vi "simulation.vi"() -> ()   [LabVIEW 2020]
uses:
  <vilib>/DAQmx/write.llb/DAQmx Write (Digital Bool 1Line 1Point).vi
  <vilib>/DAQmx/create/channels.llb/DAQmx Create Channel (DO-Digital Output).vi
  Electrical installation/Global 4.vi
  <vilib>/DAQmx/miscellaneous.llb/DAQmx Fill In Error Info.vi
  <vilib>/measure/matone.llb/Extract Single Tone Information N Chan.vi
  <vilib>/httpClient/PUTBuffer.vi
  <vilib>/httpClient/LabVIEWHTTPClient.lvlib
  <vilib>/measure/NI_MAPro.lvlib
panel:
  out "Waveform Graph 2":dynamicdata(graph)
  out "Current":dbl format="%0.3f"
  out "Current   2":dbl format="%0.3f"
  out "Buzzer":bool
  out "Flame detected":bool
  out "Fan":bool
  out "Fan Speed":dbl(knob) scale=0.0..100.0
  in  "reset switch":bool
  in  "Manual suppression":bool
  out "Fire or smoke detected":bool
  out "appended array 2":bool[](array[boolean])
  out "appended array":bool[](array[boolean])
  out "Fire Suppression":bool
  out "Smoke Detected":bool
  in  "Cluster":T1
  out "Smoke Voltage":dbl format="%0.3f"
  in  "Stop":bool
  out "Flame Voltage":dbl
  out "Temp Outside":dbl
  out "Temp Inside":dbl
  # "Smart Fire Detection And Automatic Suppression System For Electrical Distribution Boards"
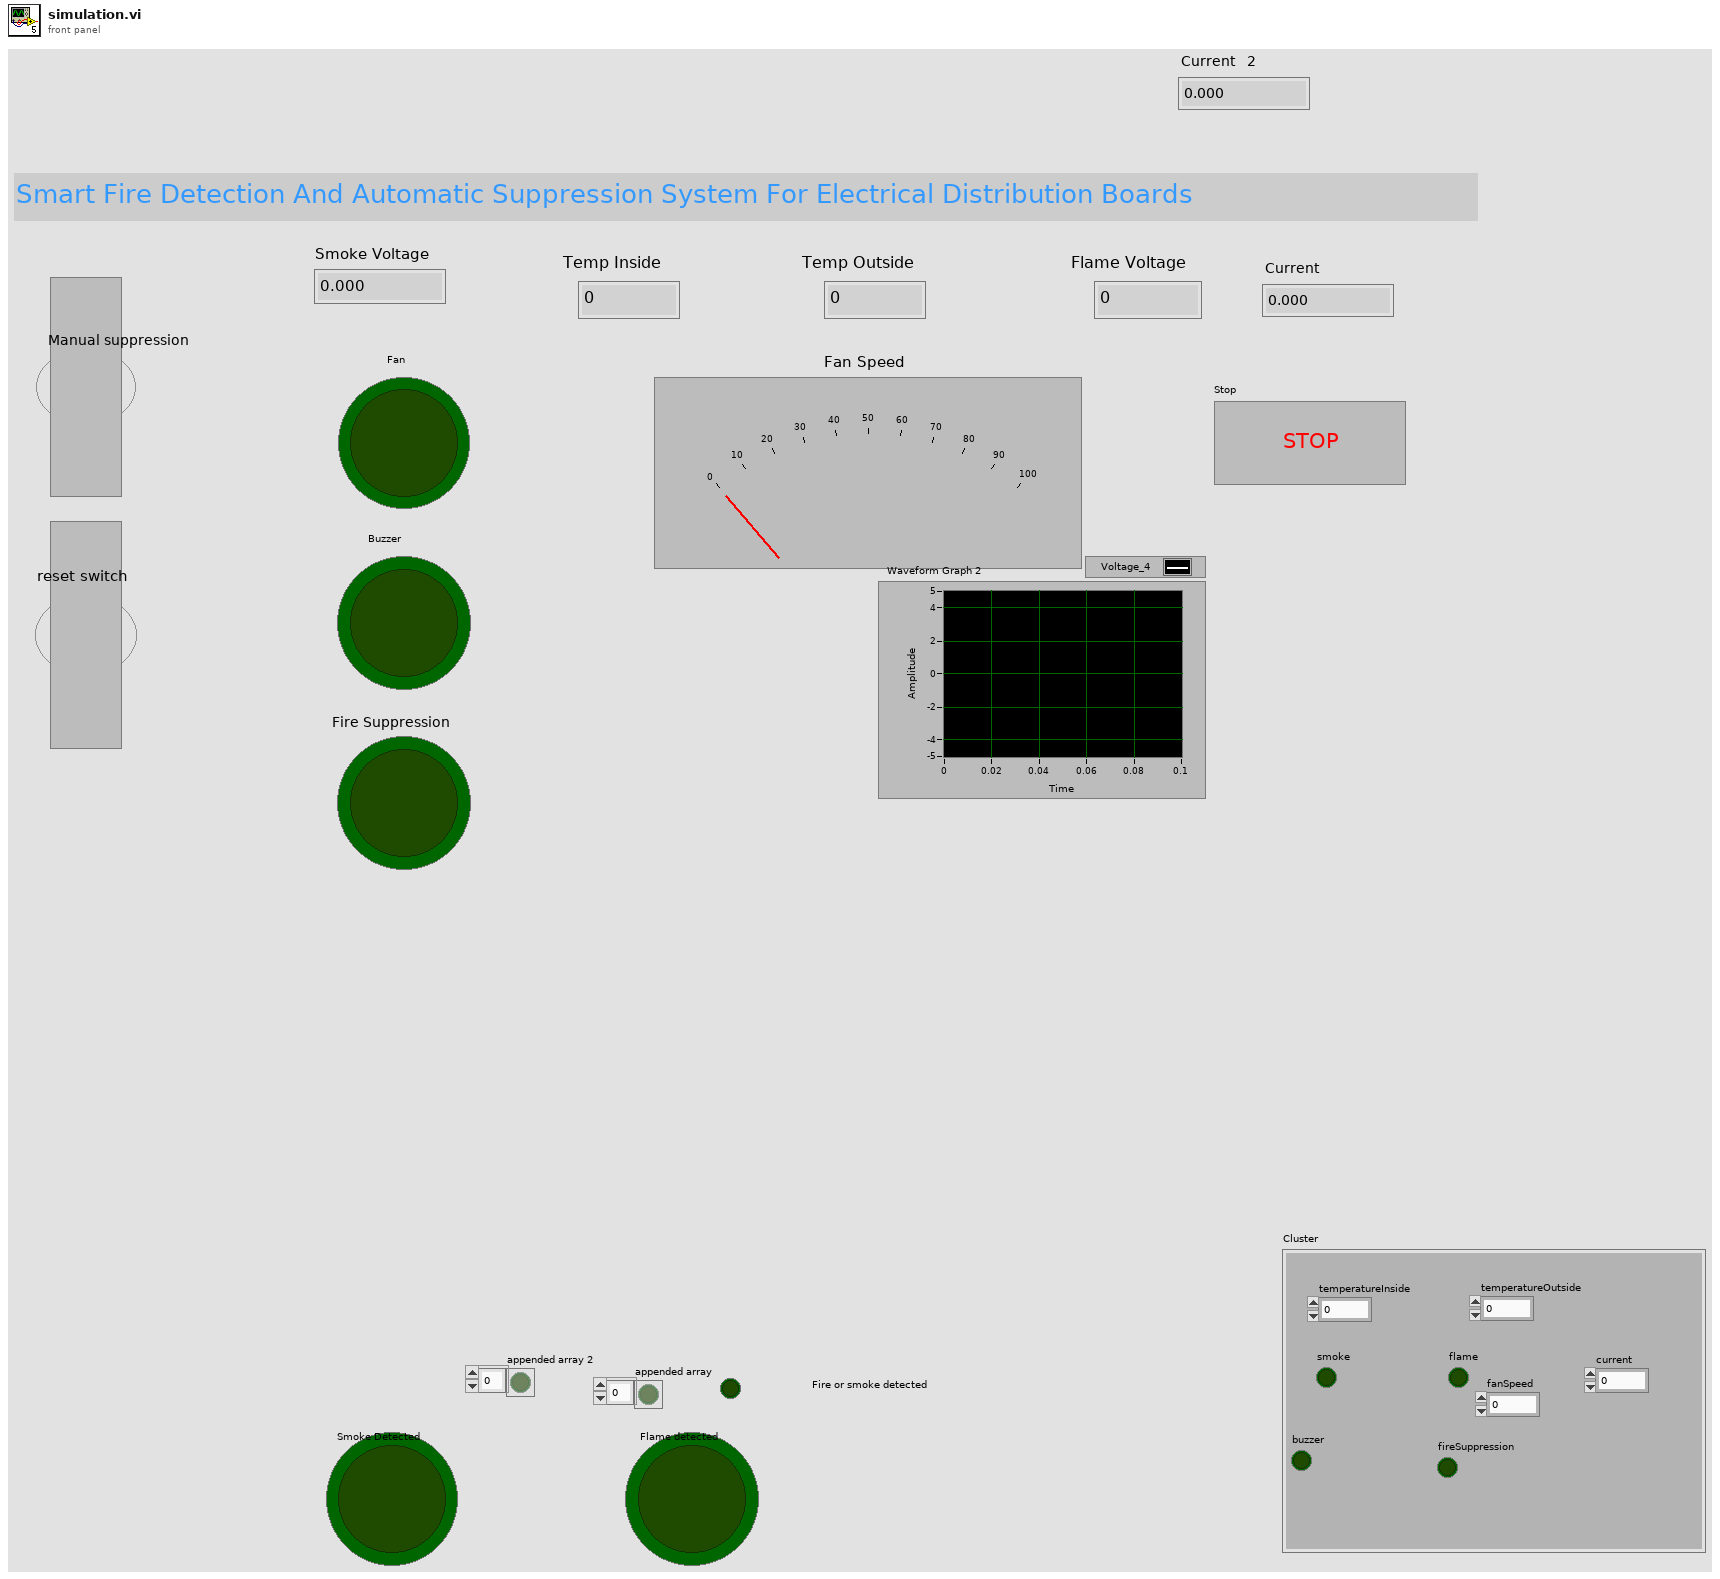
[diagram p1: front panel]
types:
  T1 = cluster{"temperatureInside":dbl, "temperatureOutside":dbl, "smoke":bool, "flame":bool, "buzzer":bool, "fireSuppression":bool, "fanSpeed":dbl, "current ":dbl}
  T2 = typedef "LabVIEWHTTPClient.lvlib/ClientHandle.ctl" = refnum<k1>
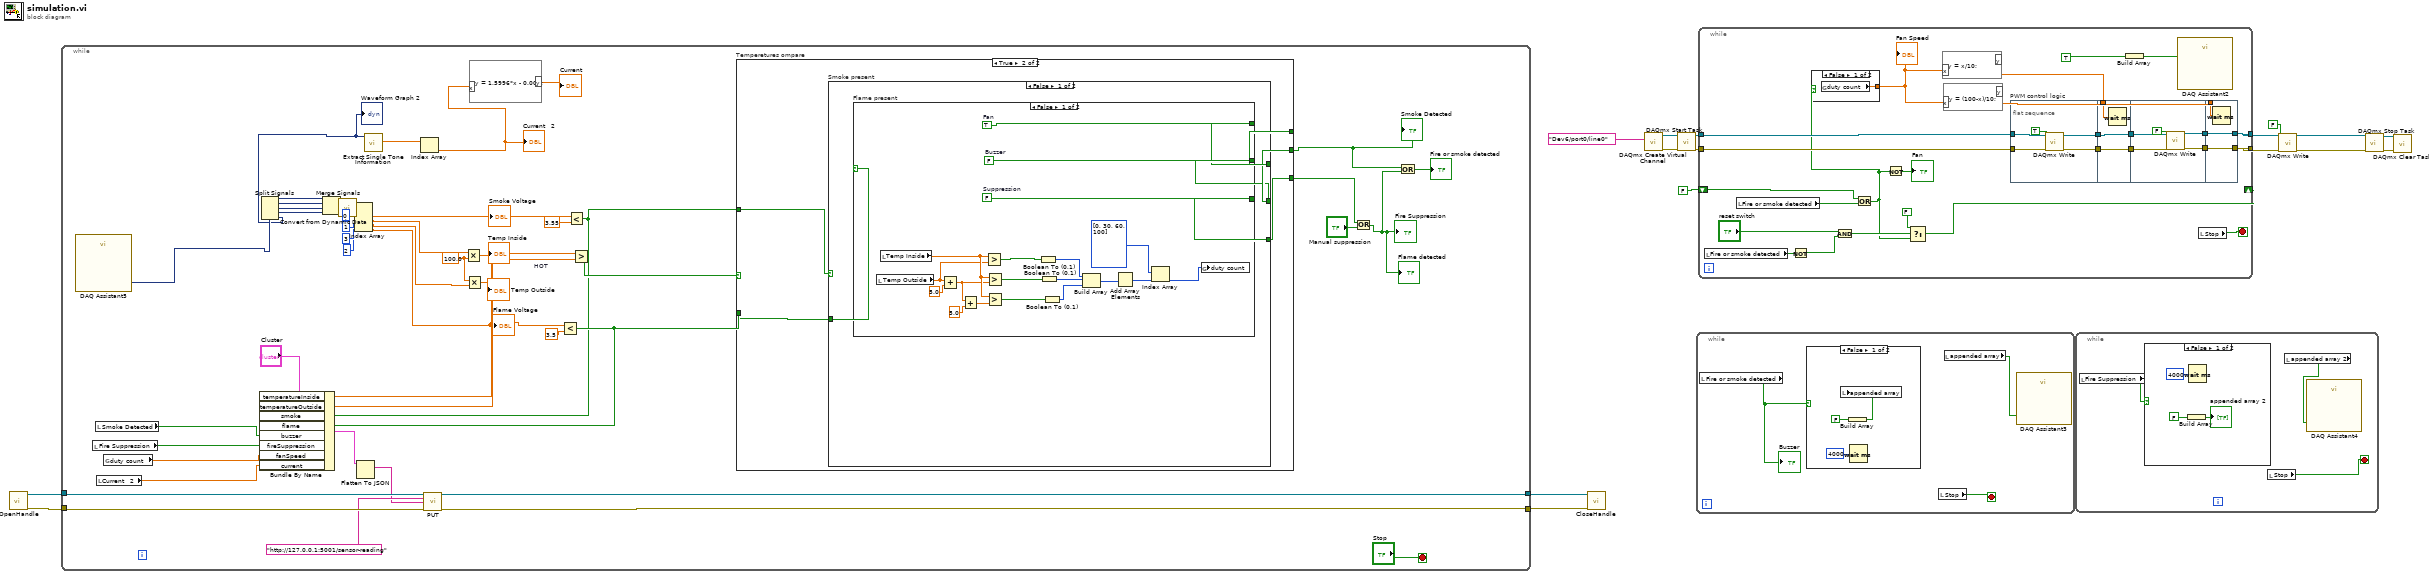
[diagram p0: block diagram]
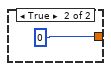
[diagram p2: hidden frame]
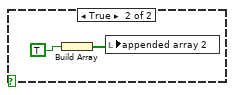
[diagram p3: hidden frame]
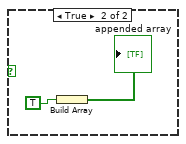
[diagram p4: hidden frame]
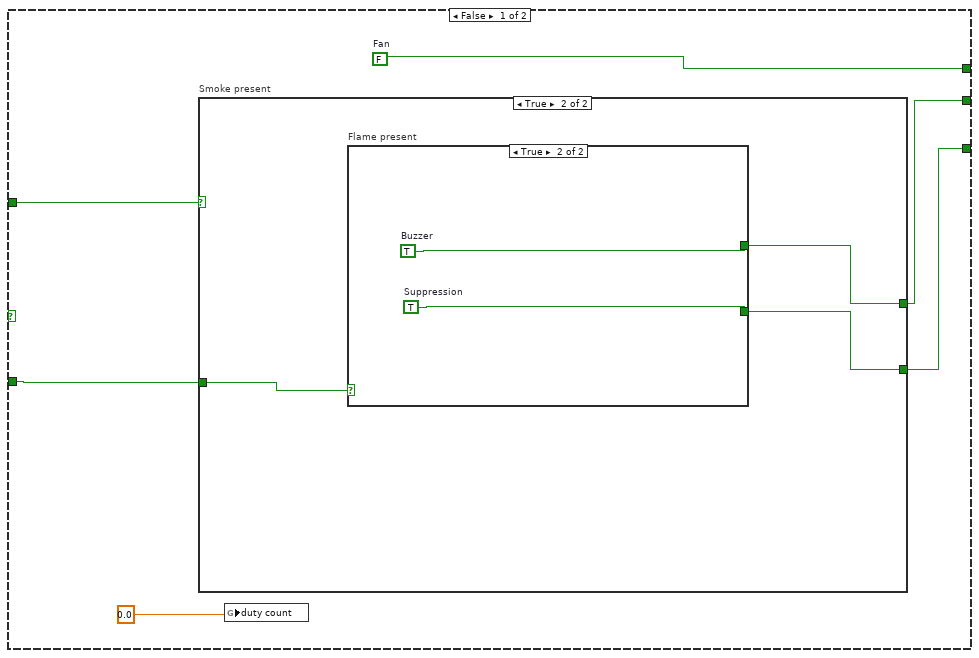
[diagram p5: hidden frame]
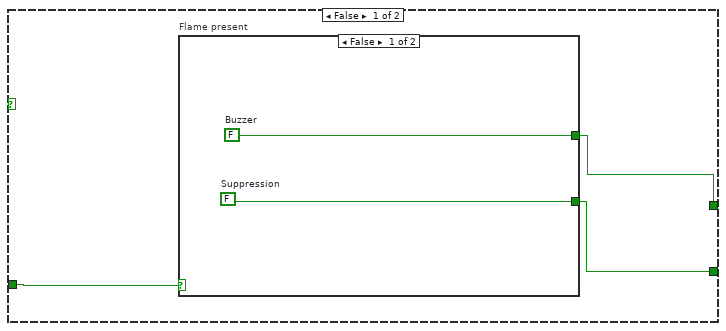
[diagram p6: hidden frame]
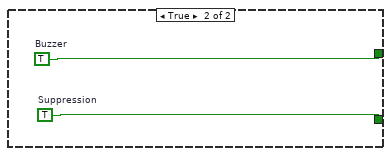
[diagram p7: hidden frame]
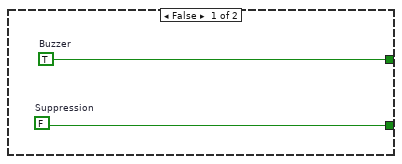
[diagram p8: hidden frame]
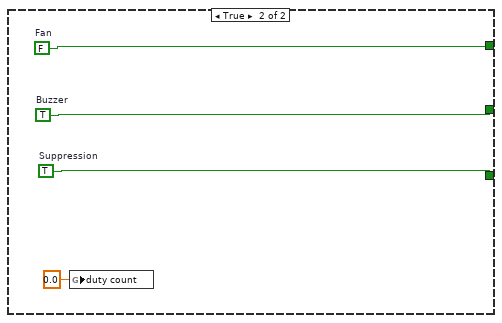
[diagram p9: hidden frame]
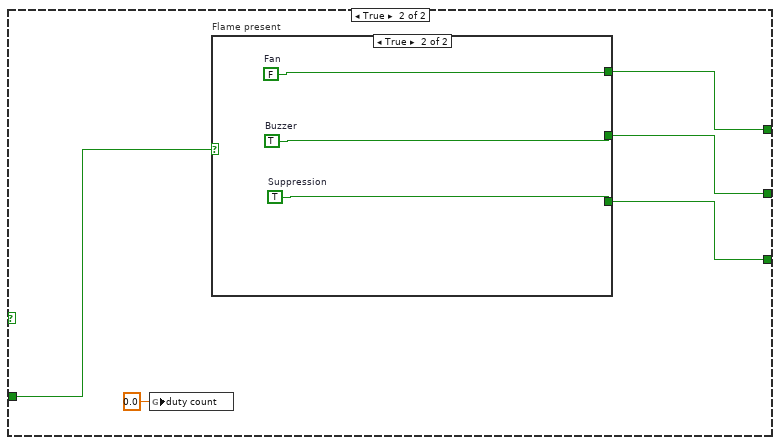
[diagram p10: hidden frame]
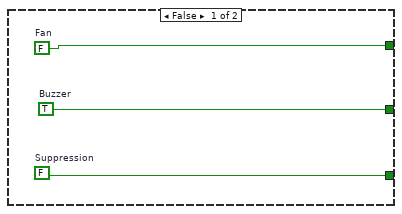
[diagram p11: hidden frame]
diagram:
  n1 = call <vilib>:"OpenHandle.vi"() -> ("client handle out"=w17:T2, "error out"=w16:errorcluster)  [unwired: 14 in]
  n2 = while {
    tunnel: w17 -> [w60]
    tunnel: w16 -> [w61]
    tunnel: [w55] -> w15
    tunnel: [w54] -> w14
    stop <- "Stop" stop-if-true
    w51 = 100.0 ("y")
    n3 = call "DAQ Assistant5"() -> ("data"=w33:dynamicdata)  [unwired: 17 in, 2 out]
    n4 = local read "Fire Suppression"() -> (w52:bool)
    n5 = local read "Smoke Detected"() -> (w53:bool)
    n6 = local read "Current   2"() -> (w37:dbl)
    n7 = global read "Global 4.vi" "duty count"() -> (w46:dbl)
    n8 = Split Signals(w33) -> (w32:dynamicdata, w31:dynamicdata, w30:dynamicdata, w29:dynamicdata, w22:dynamicdata)  [unwired: 5 in]
    "Waveform Graph 2" <- w22
    n9 = Merge Signals(w32, w31, w30, w29) -> (w28:dynamicdata)
    n10 = call "Convert from Dynamic Data"("Dynamic Data Type"=w28) -> ("Array"=w27:dbl[])  [unwired: 3 in]
    n11 = Index Array(array=w27, index #1=0 ("index"), index #2=1 ("index"), index #3=3 ("index"), index #4=2 ("index")) -> (element #1=w26:dbl, element #2=w25:dbl, element #3=w24:dbl, element #4=w23:dbl)
    "Flame Voltage" <- w23
    "Smoke Voltage" <- w26
    n12 = call-poly <vilib>:"Extract Single Tone Information.vi"("time signals in"=w22) -> ("detected amplitudes"=w34:dbl[])  [unwired: 5 in, 5 out]
    n13 = Index Array(array=w34) -> (element=w36:dbl)  [unwired: 1 in]
    "Current   2" <- w36
    n14 = Multiply(x=w25, y=w51) -> (x*y=w49:dbl)
    "Temp Inside" <- w49
    n15 = Multiply(x=w51, y=w24) -> (x*y=w50:dbl)
    "Temp Outside" <- w50
    n16 = formula code="y = 1.5996*x - 0.005;"("x"=w36) -> ("y"=→"Current":dbl)
    n17 = Less?(x=w23, y=3.5) -> (x < y?=w48:bool)
    n18 = Less?(x=w26, y=3.55) -> (x < y?=w43:bool)
    n19 = Bundle By Name(cluster="Cluster", "temperatureInside"=w49, "temperatureOutside"=w50, "smoke"=w43, "flame"=w48, "buzzer"=w53, "fireSuppression"=w52, "fanSpeed"=w46, "current"=w37) -> (w57:T1)
    n20 = Flatten To JSON(anything=w57) -> (JSON string=w58:string)  [unwired: 2 in, 1 out]
    n21 = call-poly <vilib>:"PUT.vi"("client handle"=w60, "url"="http://127.0.0.1:5001/sensor-reading", "buffer"=w58, "error in (no error)"=w61) -> ("client handle out"=w55:T2, "error out"=w54:errorcluster)  [unwired: 8 in, 2 out]
    n22 = Greater? "HOT"(x=w49, y=w50) -> (0:w62:bool)
    n23 = case "Temperetures ompare" shown="True" w62 {
      tunnel: [w68 w87] -> _
      tunnel: [w64 w86] -> w42
      tunnel: [w63 w85] -> w40
      tunnel: w43 -> [w65 w84]
      tunnel: w48 -> [w66 w83]
      frame False {
        w68 = FALSE  # Fan
        n24 = case "Smoke present" shown="True" w65 {
          tunnel: [w70 w78] -> w64
          tunnel: [w69 w77] -> w63
          tunnel: w66 -> [w71 w76]
          frame False {
            n25 = case "Flame present" shown="False" w71 {
              tunnel: [w73 w74] -> w69
              tunnel: [w72 w75] -> w70
              frame False {
                w73 = FALSE  # Suppression
                w72 = FALSE  # Buzzer
              }
              frame True {
                w74 = TRUE  # Suppression
                w75 = TRUE  # Buzzer
              }
            }
          }
          frame True {
            n26 = case "Flame present" shown="True" w76 {
              tunnel: [w80 w81] -> w77
              tunnel: [w79 w82] -> w78
              frame False {
                w80 = FALSE  # Suppression
                w79 = TRUE  # Buzzer
              }
              frame True {
                w81 = TRUE  # Suppression
                w82 = TRUE  # Buzzer
              }
            }
          }
        }
        n27 = global write "Global 4.vi" "duty count"(0.0 ("Duty cycle")) -> ()
      }
      frame True {
        n28 = case "Smoke present" shown="False" w84 {
          tunnel: [w88 w119] -> w87
          tunnel: [w90 w118] -> w86
          tunnel: [w89 w117] -> w85
          tunnel: w83 -> [w91 w115]
          frame False {
            n29 = case "Flame present" shown="False" w91 {
              tunnel: [w110 w112] -> w88
              tunnel: [w109 w113] -> w89
              tunnel: [w108 w114] -> w90
              frame False {
                w109 = FALSE  # Suppression
                w108 = FALSE  # Buzzer
                w110 = TRUE  # Fan
                n30 = local read "Temp Outside"() -> (w97:dbl)
                n31 = local read "Temp Inside"() -> (w98:dbl)
                n32 = Add(x=w97, y=5.0) -> (x+y=w96:dbl)
                n33 = Add(x=w96, y=5.0) -> (x+y=w95:dbl)
                n34 = Greater?(x=w98, y=w97) -> (0:w107:bool)
                n35 = Greater?(x=w98, y=w96) -> (0:w106:bool)
                n36 = Greater?(x=w98, y=w95) -> (0:w105:bool)
                n37 = Boolean To (0,1)(Boolean=w107) -> (0, 1=w103:i16)
                n38 = Boolean To (0,1)(Boolean=w106) -> (0, 1=w104:i16)
                n39 = Boolean To (0,1)(Boolean=w105) -> (0, 1=w102:i16)
                n40 = Build Array(w103, w104, w102) -> (w101:i16[])
                n41 = Add Array Elements(numeric array=w101) -> (sum=w100:i16)
                n42 = Index Array(array=i32[] [0, 30, 60, 100], index=w100) -> (element=w99:i32)
                n43 = global write "Global 4.vi" "duty count"(w99) -> ()
              }
              frame True {
                w113 = TRUE  # Suppression
                w114 = TRUE  # Buzzer
                w112 = FALSE  # Fan
                n44 = global write "Global 4.vi" "duty count"(0.0 ("duty count")) -> ()
              }
            }
          }
          frame True {
            n45 = global write "Global 4.vi" "duty count"(0.0 ("duty count")) -> ()
            n46 = case "Flame present" shown="True" w115 {
              tunnel: [w122 w123] -> w119
              tunnel: [w121 w124] -> w117
              tunnel: [w120 w125] -> w118
              frame False {
                w121 = FALSE  # Suppression
                w120 = TRUE  # Buzzer
                w122 = FALSE  # Fan
              }
              frame True {
                w124 = TRUE  # Suppression
                w125 = TRUE  # Buzzer
                w123 = FALSE  # Fan
              }
            }
          }
        }
      }
    }
    "Smoke Detected" <- w42
    n47 = Or(x=w40, y="Manual suppression") -> (x .or. y?=w38:bool)
    "Fire Suppression" <- w38
    "Flame detected" <- w38
    n48 = Or(x=w42, y=w38) -> (x .or. y?=→"Fire or smoke detected":bool)
  }
  n49 = call <vilib>:"CloseHandle.vi"("client handle"=w15, "error in (no error)"=w14) -> ()  [unwired: 13 in, 1 out]
  n50 = call-poly <vilib>:"DAQmx Create Virtual Channel.vi"("lines"=tag "Dev6/port0/line0") -> ("task out"=w13:refnum<k21>, "error out"=w12:errorcluster)  [unwired: 13 in]
  n51 = call <vilib>:"DAQmx Start Task.vi"("task/channels in"=w13, "error in"=w12) -> ("task out"=w11:refnum<k21>, "error out"=w10:errorcluster)  [unwired: 12 in]
  n52 = while {
    stop <- w128 stop-if-true
    n53 = local read "Fire or smoke detected"() -> (w126:bool)
    "Buzzer" <- w126
    n54 = case shown="False" w126 {
      frame False {
        n55 = Build Array(FALSE) -> (w130:bool[])
        n56 = local write "appended array"(w130) -> ()
        n57 = Wait (ms)(milliseconds to wait=u32 4000) -> ()  [unwired: 1 out]
      }
      frame True {
        n58 = Build Array(TRUE) -> (→"appended array":bool[])
      }
    }
    n59 = local read "Stop"() -> (w128:bool)
    n60 = local read "appended array"() -> (w127:bool[])
    n61 = call "DAQ Assistant3"("data"=w127) -> ()  [unwired: 17 in, 2 out]
  }
  n62 = while {
    tunnel: w11 -> [w159]
    tunnel: w10 -> [w158]
    tunnel: [w151] -> w5
    tunnel: [w150] -> w4
    shift-right: [w136] -> _
    shift-left: FALSE ("Fire or smoke detected") -> [w144]
    stop <- w145 stop-if-true
    n63 = local read "Fire or smoke detected"() -> (w142:bool)
    n64 = local read "Fire or smoke detected"() -> (w143:bool)
    n65 = Not(x=w142) -> (.not. x?=w141:bool)
    n66 = And(x="reset switch", y=w141) -> (x .and. y?=w137:bool)
    n67 = Or(x=w144, y=w143) -> (x .or. y?=w135:bool)
    n68 = case shown="False" w135 {
      tunnel: [w160 0] -> w139
      frame False {
        n69 = global read "Global 4.vi" "duty count"() -> (w160:dbl)
      }
      frame True {
      }
    }
    "Fan Speed" <- w139
    n70 = Not(x=w135) -> (.not. x?=→"Fan":bool)
    n71 = Select(t=FALSE, s=w137, f=w135) -> (s? t:f=w136:bool)
    n72 = formula code="y = x/10;"("x"=w139) -> ("y"=w148:dbl)
    n73 = formula code="y = (100-x)/10;"("x"=w139) -> ("y"=w147:dbl)
    n74 = flat-sequence "PWM control logic" {
      tunnel: w159 -> [w166]
      tunnel: w158 -> [w165]
      tunnel: [w164] -> w157
      tunnel: [w163] -> w154
      tunnel: w157 -> [w169]
      tunnel: [w169] -> w156
      tunnel: [w168] -> w155
      tunnel: w154 -> [w168]
      tunnel: w148 -> [w167]
      tunnel: w156 -> [w174]
      tunnel: w155 -> [w173]
      tunnel: [w171] -> w153
      tunnel: [w170] -> w152
      tunnel: w153 -> [w177]
      tunnel: w152 -> [w176]
      tunnel: [w177] -> w151
      tunnel: [w176] -> w150
      tunnel: w147 -> [w175]
      frame #0 {
        n75 = call-poly <vilib>:"DAQmx Write.vi"("task/channels in"=w166, "data"=TRUE, "error in"=w165) -> ("task out"=w164:refnum<k21>, "error out"=w163:errorcluster)  [unwired: 10 in, 1 out]
      }
      frame #1 {
        n76 = Wait (ms)(milliseconds to wait=w167) -> ()  [unwired: 1 out]
      }
      frame #2 {
        n77 = call-poly <vilib>:"DAQmx Write.vi"("task/channels in"=w174, "data"=FALSE, "error in"=w173) -> ("task out"=w171:refnum<k21>, "error out"=w170:errorcluster)  [unwired: 10 in, 1 out]
      }
      frame #3 {
        n78 = Wait (ms)(milliseconds to wait=w175) -> ()  [unwired: 1 out]
      }
    }
    n79 = Build Array(TRUE) -> (w149:bool[])
    n80 = call "DAQ Assistant2"("data"=w149) -> ()  [unwired: 17 in, 2 out]
    n81 = local read "Stop"() -> (w145:bool)
  }
  n82 = while {
    stop <- w180 stop-if-true
    n83 = local read "Fire Suppression"() -> (w179:bool)
    n84 = case shown="False" w179 {
      frame False {
        n85 = Build Array(FALSE) -> (→"appended array 2":bool[])
        n86 = Wait (ms)(milliseconds to wait=u32 4000) -> ()  [unwired: 1 out]
      }
      frame True {
        n87 = Build Array(TRUE) -> (w184:bool[])
        n88 = local write "appended array 2"(w184) -> ()
      }
    }
    n89 = local read "Stop"() -> (w180:bool)
    n90 = local read "appended array 2"() -> (w178:bool[])
    n91 = call "DAQ Assistant4"("data"=w178) -> ()  [unwired: 17 in, 2 out]
  }
  n92 = call-poly <vilib>:"DAQmx Write.vi"("task/channels in"=w5, "data"=FALSE, "error in"=w4) -> ("task out"=w7:refnum<k21>, "error out"=w6:errorcluster)  [unwired: 10 in, 1 out]
  n93 = call <vilib>:"DAQmx Stop Task.vi"("task/channels in"=w7, "error in"=w6) -> ("task out"=w9:refnum<k21>, "error out"=w8:errorcluster)  [unwired: 12 in]
  n94 = call <vilib>:"DAQmx Clear Task.vi"("task in"=w9, "error in"=w8) -> ()  [unwired: 13 in, 1 out]
